vi "User Variable.vi"(6 "size/resize (0-10001)":i32=1, 7 "unit (optional)":string, 8 "error in (no error)":errorcluster, 9 "variable name (\"UVAR1\") (max 6 chars)":string="UVAR1", 10 "operation":i32(slide) max=4 scale=0.0..4.0, 11 "VISA session":refnum<visa-resource-name>) -> (0 "error out":errorcluster, 2 "currently defined user variables":string, 3 "VISA resource name out":refnum<visa-resource-name>)   [LabVIEW 2016, in "Agilent 415X Series.lvlib"]
doc: "In this VI, you define/delete/list user variables. For details about user functions, refer to \"User Variable\" in Chapter 6 of User's Dictionary Reference.\n\n* This VI does NOT perform any error checking on the control settings. That is, this VI does not check the length of UNIT or NAME. Entering a string longer than allowed will cause an error to be placed in the instrument's error queue. To read the error queue, run HP415xA Sys-Report Error.vi."
uses:
  Agilent 415X Series.lvlib
panel:
  # "* 0 = auto-size"
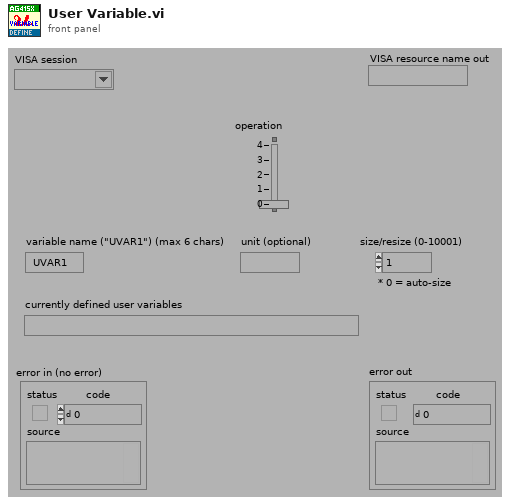
[diagram p1: front panel]
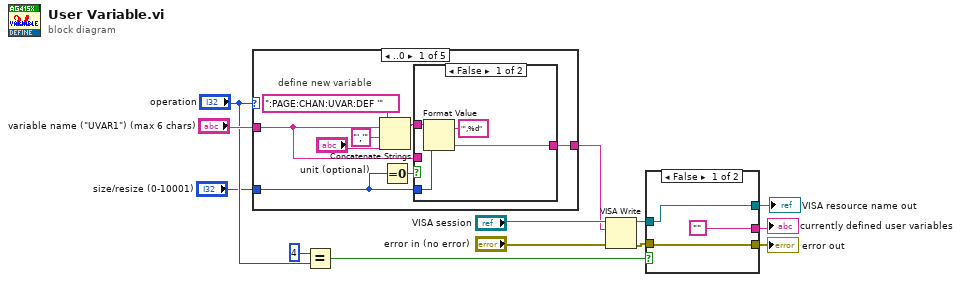
[diagram p0: block diagram]
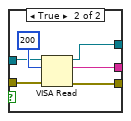
[diagram p2: hidden frame]
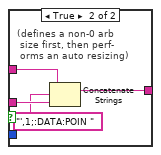
[diagram p3: hidden frame]
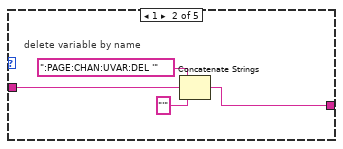
[diagram p4: hidden frame]
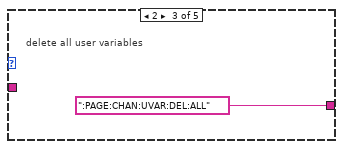
[diagram p5: hidden frame]
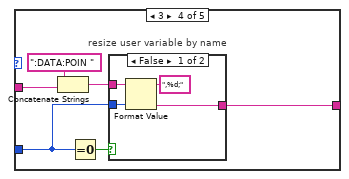
[diagram p6: hidden frame]
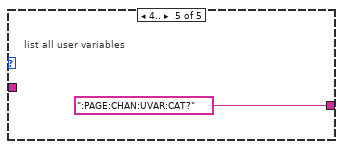
[diagram p8: hidden frame]
diagram:
  n1 = case shown="..0" "operation" {
    tunnel: [w17 w32 ":PAGE:CHAN:UVAR:DEL:ALL" w36 ":PAGE:CHAN:UVAR:CAT?"] -> w10
    tunnel: "variable name (\"UVAR1\") (max 6 chars)" -> [w14 w30 _ w40 _]
    tunnel: "size/resize (0-10001)" -> [w15 _ _ w35 _]
    frame ..0 {
      # "define new variable"
      n2 = Concatenate Strings(":PAGE:CHAN:UVAR:DEF '", w14, "','", "unit (optional)") -> (w18:string)
      n3 = Equal To 0?(x=w15) -> (x = 0?=w16:bool)
      n4 = case shown="False" w16 {
        tunnel: w18 -> [w24 w28]
        tunnel: [w23 w29] -> w17
        tunnel: w15 -> [w22 _]
        tunnel: w14 -> [_ w27]
        frame False {
          n5 = Format Value(string ("")=w24, format string="',%d", value (0)=w22) -> (output string=w23:string)
        }
        frame True {
          # "(defines a non-0 arb\n size first, then perf-\n orms an auto resizing)"
          n6 = Concatenate Strings(w28, "',1;:DATA:POIN ", w27) -> (w29:string)
        }
      }
    }
    frame 1 {
      # "delete variable by name"
      n7 = Concatenate Strings(":PAGE:CHAN:UVAR:DEL '", w30, "'") -> (w32:string)
    }
    frame 2 {
      # "delete all user variables"
    }
    frame 3 {
      # "resize user variable by name"
      n8 = Concatenate Strings(":DATA:POIN ", w40) -> (w38:string)
      n9 = Equal To 0?(x=w35) -> (x = 0?=w37:bool)
      n10 = case shown="False" w37 {
        tunnel: w38 -> [w43 w45]
        tunnel: [w42 w45] -> w36
        tunnel: w35 -> [w41 _]
        frame False {
          n11 = Format Value(string ("")=w43, format string=",%d;", value (0)=w41) -> (output string=w42:string)
        }
        frame True {
          # "auto-resizing"
        }
      }
    }
    frame 4.. {
      # "list all user variables"
    }
  }
  n12 = Equal?(x=4, y="operation") -> (x = y?=w4:bool)
  n13 = VISA Write(VISA resource name="VISA session", write buffer=w10, error in (no error)="error in (no error)") -> (VISA resource name out=w9:refnum<visa-resource-name>, error out=w8:errorcluster)  [unwired: 1 out]
  n14 = case shown="False" w4 {
    tunnel: w9 -> [w47 w54]
    tunnel: w8 -> [w48 w53]
    tunnel: [w48 w52] -> w7
    tunnel: ["" ("Empty String Constant") w51] -> w6
    tunnel: [w47 w50] -> w1
    frame False {
    }
    frame True {
      n15 = VISA Read(VISA resource name=w54, byte count=u32 200, error in (no error)=w53) -> (VISA resource name out=w50:refnum<visa-resource-name>, read buffer=w51:string, error out=w52:errorcluster)  [unwired: 1 out]
    }
  }
  "error out" <- w7
  "currently defined user variables" <- w6
  "VISA resource name out" <- w1
